vi "GetText.vi"(8 "error in":errorcluster, 11 "group in":refnum<class "Group.lvclass">) -> (0 "error out":errorcluster, 1 "additional text":string, 2 "text":string, 3 "group out":refnum<class "Group.lvclass">, 4 "glyph":string)   [LabVIEW 2015, in "Group.lvclass"]
uses:
  Group.lvclass
  Group.lvclass/Group.ctl
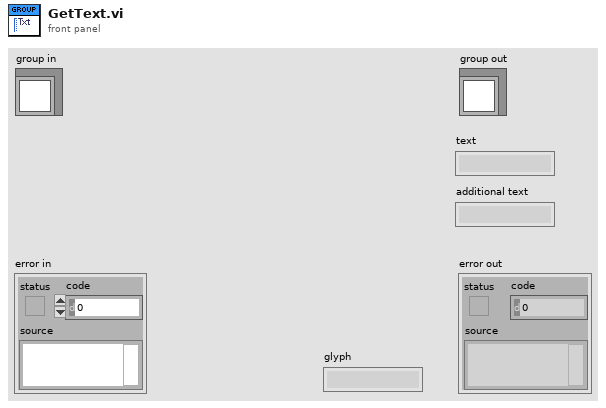
[diagram p1: front panel]
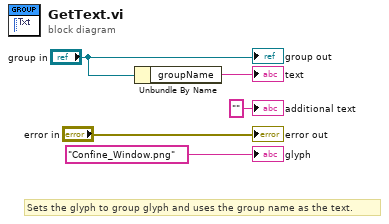
[diagram p0: block diagram]
diagram:
  # "Sets the glyph to group glyph and uses the group name as the text."
  n1 = Unbundle By Name("group in") -> ("groupName"=→"text":string)
  "error out" <- "error in"
  "group out" <- "group in"
  "additional text" <- "" ("additional text")
  "glyph" <- "Confine_Window.png" ("glyph")
